vi "GTH-V2.ADC.vi"(6 "Signal Filter":T2={"Type"=enum."None", "Freq"=10000.0, "FreqB"=100.0}, 7 "Calibration_Para":dbl[][](array[numeric]), 8 "Error In":errorcluster caption="错误输入", 9 "ADC_Para":T1={"Points(X*5k)"=10, "SampleRate"=250000, "Rate"=1.0} {"Rate" min=0.01 max=100.0; "SampleRate" min=1000 max=250000 step=1000; "Points(X*5k)" min=1 max=100}, 10 "Channel":enum16{"ChanA1", "ChanA2", "ChanB1", "ChanB2"}(ring), 11 "VISA资源输入":refnum<visa-resource-name>="USB0::0x3323::0x0001::48E3845A3737::RAW") -> (0 "Error Out":errorcluster caption="错误输出", 1 "波形图":waveform(dbl)(graph), 2 "DataOut":T3={"频率"=37677.78979590854, "峰峰值"=0.1934065934065934, "均值（直流）"=-0.005379487179487172, "均方根"=0.04788898808560139, "正峰"=0.093, "反峰"=-0.10040659340659341, "幅值"=0.007320515046354128, "均方根(AC)"=0.047585883385186885} {"幅值" format="%#_8f"; "均值（直流）" format="%#_8f"}, 3 "OK?":bool=TRUE)   [LabVIEW 2012, in "Lib_UEL.ATE.lvlib" / "STM32-CoreBD.lvlib"]
uses:
  STM32-CoreBD.lvlib
  <vilib>/measure/madcrms.llb/Basic Averaged DC-RMS for 1 Chan.vi
  <vilib>/measure/NI_MAPro.lvlib
panel:
  # "Version History\nV1.0.0, 2015-8-10, GTH-V2初始版本.\nV1.1.0, 2015-10-9, ADC_Para增加Rate参数."
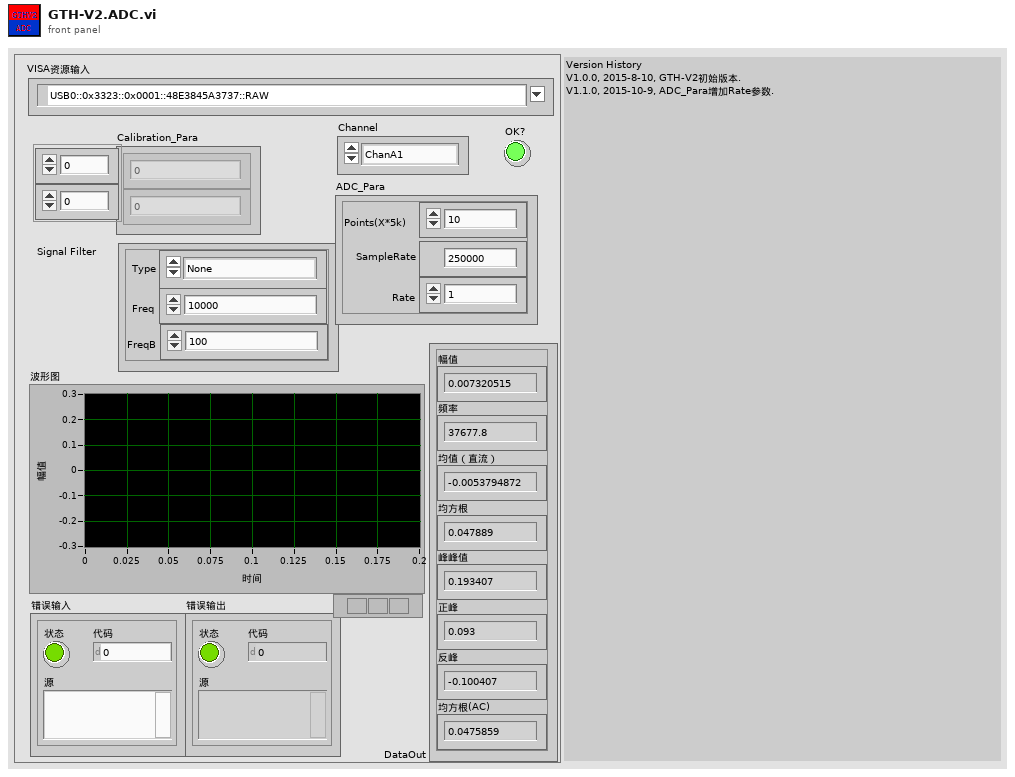
[diagram p1: front panel]
types:
  T1 = cluster{"Points(X*5k)":u8, "SampleRate":u32, "Rate":dbl}
  T2 = cluster{"Type":enum16{"None", "Low Pass", "High Pass", "Band Pass"}, "Freq":dbl, "FreqB":dbl}
  T3 = cluster{"频率":dbl, "峰峰值":dbl, "均值（直流）":dbl, "均方根":dbl, "正峰":dbl, "反峰":dbl, "幅值":dbl, "均方根(AC)":dbl}
  T4 = enum16{"Read_Version", "Read_PID", "Read_CalibrationInfo", "Read_C_Value_ADC_ChanA", "Read_C_Value_ADC_ChanB", "Read_C_Value_Current", "Read_C_Value_DAC", "Write_CalibrationInfo", "Write_C_Value_ADC_ChanA", "Write_C_Value_ADC_ChanB", "Write_C_Value_Current", "Write_C_Value_DAC"}
  T5 = enum16{"None", "Low Pass", "High Pass", "Band Pass"}
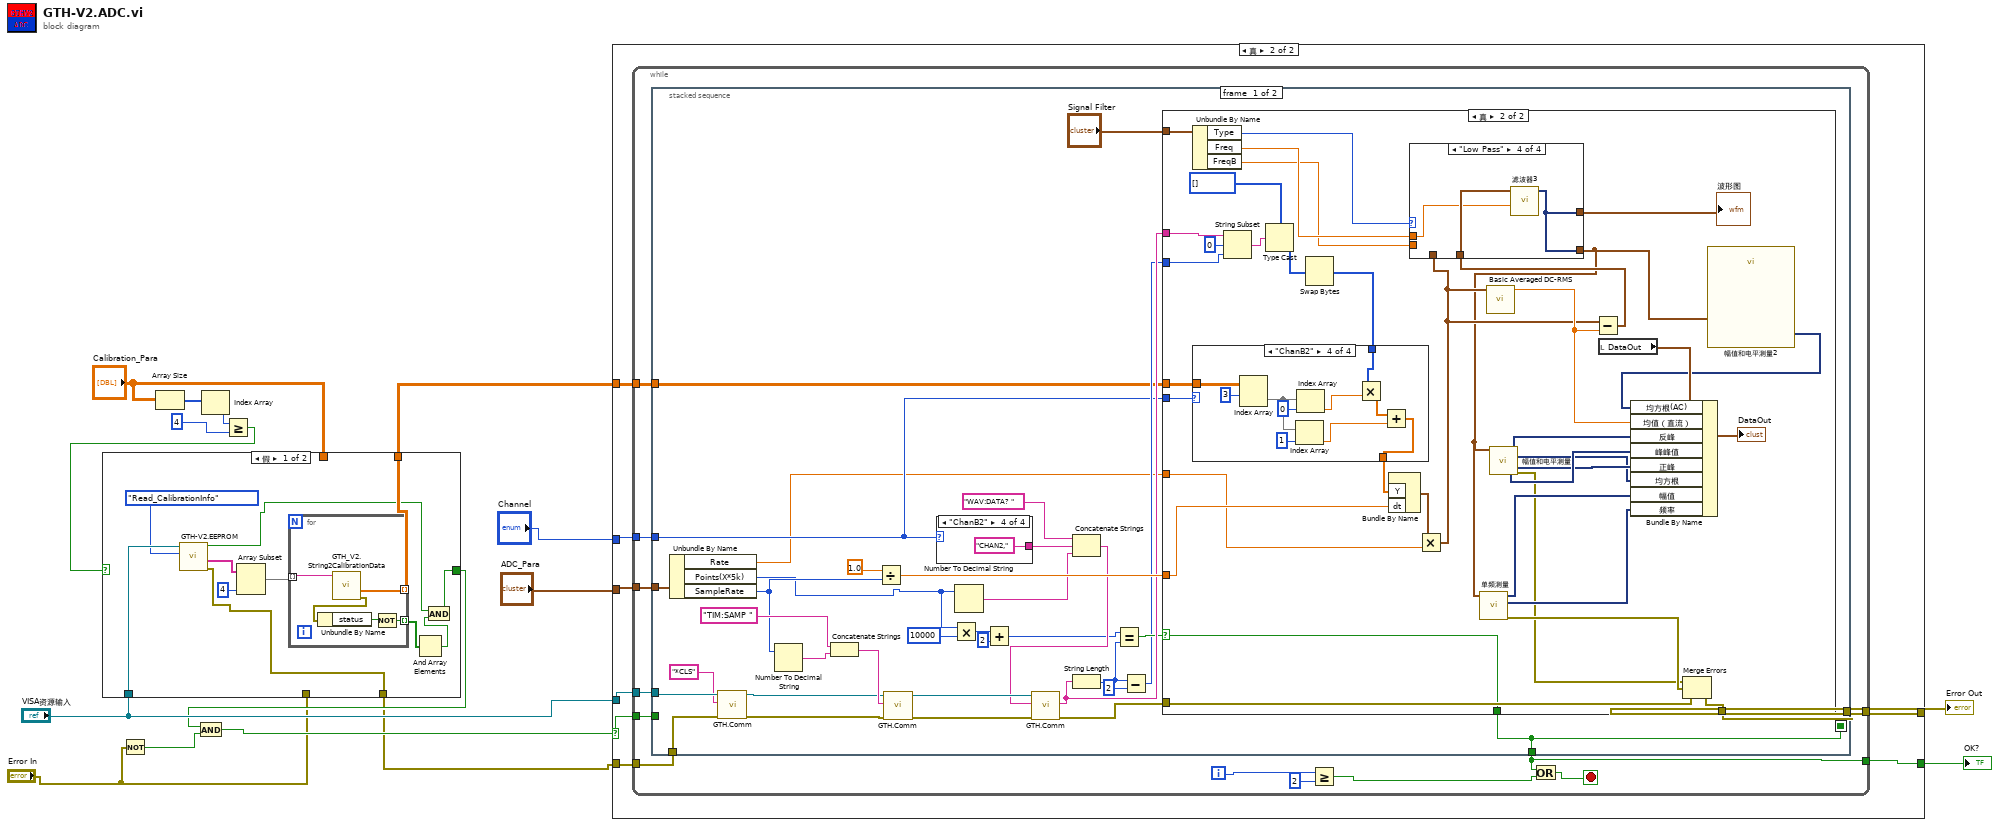
[diagram p0: block diagram]
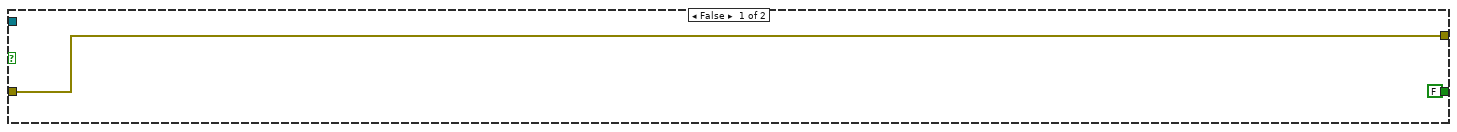
[diagram p3: hidden frame]
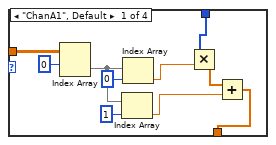
[diagram p5: hidden frame]
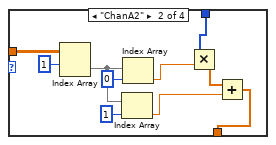
[diagram p6: hidden frame]
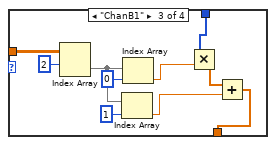
[diagram p7: hidden frame]
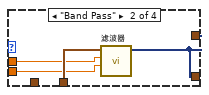
[diagram p9: hidden frame]
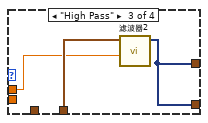
[diagram p10: hidden frame]
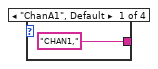
[diagram p11: hidden frame]
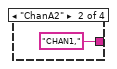
[diagram p12: hidden frame]
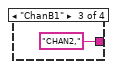
[diagram p13: hidden frame]
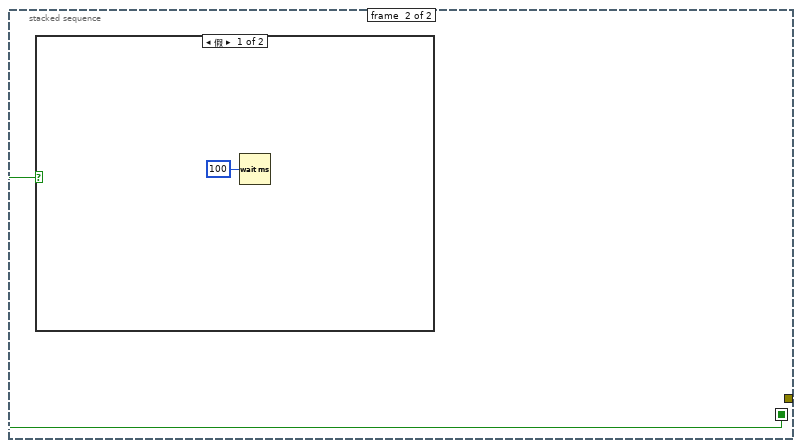
[diagram p14: hidden frame]
diagram:
  n1 = Not(x="Error In") -> (.not. x?=w10:bool)
  n2 = Array Size(array="Calibration_Para") -> (size(s)=w6:i32[])
  n3 = Index Array(array=w6) -> (element=w5:i32)  [unwired: 1 in]
  n4 = Greater Or Equal?(x=w5, y=4) -> (x >= y?=w4:bool)
  n5 = case shown="假" w4 {
    selector: w4 -> [_ w34]
    tunnel: [w22 w35] -> w9
    tunnel: "Calibration_Para" -> [_ w35]
    tunnel: "VISA资源输入" -> [w27 _]
    tunnel: [w20 w34] -> w3
    tunnel: [w19 w33] -> w2
    tunnel: "Error In" -> [_ w33]
    frame False {
      n6 = call "GTH-V2.EEPROM.vi"("CMD"=T4."Read_CalibrationInfo", "VISA资源输入"=w27) -> ("Error Out"=w19:errorcluster, "Calibration_Value_Out"=w25:string[], "OK?"=w21:bool)  [unwired: 6 in, 1 out]
      n7 = Array Subset(array=w25, length=4 ("长度")) -> (w23:string[])  [unwired: 1 in]
      n8 = for {
        tunnel: w23 -> [w32] mode=indexing
        tunnel: [w31] -> w22 mode=indexing
        tunnel: [w28] -> w18 mode=indexing
        n9 = call "GTH_V2.String2CalibrationData.vi"("String"=w32) -> ("错误输出"=w29:errorcluster, "Para"=w31:dbl[])  [unwired: 5 in, 4 out]
        n10 = Unbundle By Name(w29) -> ("status"=w30:bool)
        n11 = Not(x=w30) -> (.not. x?=w28:bool)
      }
      n12 = And Array Elements(Boolean array=w18) -> (logical AND=w17:bool)
      n13 = And(x=w21, y=w17) -> (x .and. y?=w20:bool)
    }
    frame True {
    }
  }
  n14 = And(x=w3, y=w10) -> (x .and. y?=w12:bool)
  n15 = case shown="真" w12 {
    selector: w12 -> [_ w43]
    tunnel: [w36 w45] -> w16
    tunnel: "VISA资源输入" -> [_ w44]
    tunnel: [FALSE w42] -> w15
    tunnel: "ADC_Para" -> [_ w41]
    tunnel: "Channel" -> [_ w40]
    tunnel: w2 -> [w36 w38]
    tunnel: w9 -> [_ w39]
    frame False {
    }
    frame True {
      n16 = while {
        tunnel: [w54] -> w45
        tunnel: w44 -> [w57]
        tunnel: w43 -> [w56]
        tunnel: [w50] -> w42
        tunnel: w41 -> [w49]
        tunnel: w40 -> [w48]
        tunnel: w39 -> [w47]
        tunnel: w38 -> [w46]
        i -> [w53]
        stop <- w55 stop-if-true
        n17 = stacked-sequence {
          seq-local: [w66 _] -> [_ w186]
          tunnel: w57 -> [w88 _]
          tunnel: w56 -> [_ _]
          tunnel: [w67 _] -> w54
          tunnel: [w66 _] -> w50
          tunnel: w49 -> [w64 _]
          tunnel: w48 -> [w61 _]
          tunnel: w47 -> [w60 _]
          tunnel: w46 -> [w59 _]
          frame #0 {
            n18 = Unbundle By Name(w64) -> ("Rate"=w58:dbl, "Points(X*5k)"=w62:u8, "SampleRate"=w63:u32)
            n19 = call "GTH.Comm.vi"("Error In"=w59, "SCPI CMD"="*CLS" ("字符串"), "USB Port In"=w88) -> ("Error Out"=w82:errorcluster, "USB Port Out"=w83:refnum<visa-resource-name>)  [unwired: 3 in, 4 out]
            n20 = Number To Decimal String(number=w63) -> (decimal integer string=w85:string)  [unwired: 1 in]
            n21 = Concatenate Strings("TIM:SAMP " ("字符串"), w85) -> (w84:string)
            n22 = Divide(x=1.0 ("y"), y=w63) -> (x/y=w89:dbl)
            n23 = call "GTH.Comm.vi"("Error In"=w82, "SCPI CMD"=w84, "USB Port In"=w83) -> ("Error Out"=w79:errorcluster, "USB Port Out"=w80:refnum<visa-resource-name>)  [unwired: 3 in, 4 out]
            n24 = case shown="\"ChanB2\"" w61 {
              tunnel: ["CHAN1," ("字符串") "CHAN1," ("字符串") "CHAN2," ("字符串") "CHAN2," ("字符串")] -> w91
              frame "ChanA1", Default {
              }
              frame "ChanA2" {
              }
              frame "ChanB1" {
              }
              frame "ChanB2" {
              }
            }
            n25 = Multiply(x=w62, y=u32 10000) -> (x*y=w75:u32)
            n26 = Number To Decimal String(number=w62) -> (decimal integer string=w81:string)  [unwired: 1 in]
            n27 = Add(x=w75, y=u32 2) -> (x+y=w72:u32)
            n28 = Concatenate Strings("WAV:DATA? " ("字符串"), w91, w81) -> (w78:string)
            n29 = call "GTH.Comm.vi"("Error In"=w79, "SCPI CMD"=w78, "USB Port In"=w80) -> ("Error Out"=w77:errorcluster, "Return"=w73:string)  [unwired: 3 in, 4 out]
            n30 = String Length(string=w73) -> (length=w70:i32)
            n31 = Equal?(x=w72, y=w70) -> (x = y?=w71:bool)
            n32 = Subtract(x=w70, y=2) -> (x-y=w68:i32)
            n33 = case shown="真" w71 {
              selector: w71 -> [w93 w115]
              tunnel: w89 -> [_ w128]
              tunnel: [w94 w122] -> w67
              tunnel: w77 -> [w94 w120]
              tunnel: w73 -> [_ w118]
              tunnel: w68 -> [_ w116]
              tunnel: [w93 w115] -> w66
              tunnel: "Signal Filter" -> [_ w108]
              tunnel: w61 -> [_ w103]
              tunnel: w60 -> [_ w102]
              tunnel: w58 -> [_ w99]
              frame False {
              }
              frame True {
                n34 = Unbundle By Name(w108) -> ("Type"=w107:T5, "Freq"=w104:dbl, "FreqB"=w95:dbl)
                n35 = String Subset(string=w118, offset (0)=0 ("偏移量(0)"), length (rest)=w116) -> (substring=w119:string)
                n36 = Type Cast(type=u16[] [], x=w119) -> (*(type *) &x=w129:u16[])
                n37 = Swap Bytes(anything=w129) -> (byte swapped=w100:u16[])
                n38 = case shown="\"ChanB2\"" w103 {
                  tunnel: w102 -> [w140 w150 w160 w170]
                  tunnel: w100 -> [w138 w148 w158 w168]
                  tunnel: [w136 w146 w156 w166] -> w101
                  frame "ChanA1", Default {
                    n39 = Index Array(array=w140, index (row)=0 ("索引")) -> (element=w135:dbl[])  [unwired: 1 in]
                    n40 = Index Array(array=w135, index=1 ("索引")) -> (element=w131:dbl)
                    n41 = Index Array(array=w135, index=0 ("索引")) -> (element=w132:dbl)
                    n42 = Multiply(x=w138, y=w132) -> (x*y=w137:dbl[])
                    n43 = Add(x=w137, y=w131) -> (x+y=w136:dbl[])
                  }
                  frame "ChanA2" {
                    n44 = Index Array(array=w150, index (row)=1 ("索引")) -> (element=w145:dbl[])  [unwired: 1 in]
                    n45 = Index Array(array=w145, index=1 ("索引")) -> (element=w141:dbl)
                    n46 = Index Array(array=w145, index=0 ("索引")) -> (element=w142:dbl)
                    n47 = Multiply(x=w148, y=w142) -> (x*y=w147:dbl[])
                    n48 = Add(x=w147, y=w141) -> (x+y=w146:dbl[])
                  }
                  frame "ChanB1" {
                    n49 = Index Array(array=w160, index (row)=2 ("索引")) -> (element=w155:dbl[])  [unwired: 1 in]
                    n50 = Index Array(array=w155, index=1 ("索引")) -> (element=w151:dbl)
                    n51 = Index Array(array=w155, index=0 ("索引")) -> (element=w152:dbl)
                    n52 = Multiply(x=w158, y=w152) -> (x*y=w157:dbl[])
                    n53 = Add(x=w157, y=w151) -> (x+y=w156:dbl[])
                  }
                  frame "ChanB2" {
                    n54 = Index Array(array=w170, index (row)=3 ("索引")) -> (element=w165:dbl[])  [unwired: 1 in]
                    n55 = Index Array(array=w165, index=1 ("索引")) -> (element=w161:dbl)
                    n56 = Index Array(array=w165, index=0 ("索引")) -> (element=w162:dbl)
                    n57 = Multiply(x=w168, y=w162) -> (x*y=w167:dbl[])
                    n58 = Add(x=w167, y=w161) -> (x+y=w166:dbl[])
                  }
                }
                n59 = Bundle By Name("Y"=w101, "dt"=w128) -> (w98:waveform(dbl))  [unwired: 1 in]
                n60 = Multiply(x=w98, y=w99) -> (x*y=w97:waveform(dbl))
                n61 = call-poly <vilib>:"Basic Averaged DC-RMS.vi"("signal in"=w97) -> ("DC value"=w121:dbl)  [unwired: 7 in, 3 out]
                n62 = Subtract(x=w97, y=w121) -> (x-y=w105:waveform(dbl))
                n63 = case shown="\"Low Pass\"" w107 {
                  tunnel: [w171 w174 w176 w179] -> w106
                  tunnel: w97 -> [w171 _ _ _]
                  tunnel: [w171 w174 w176 w179] -> w96
                  tunnel: w105 -> [_ w175 w178 w181]
                  tunnel: w104 -> [_ w173 w177 w180]
                  tunnel: w95 -> [_ w172 _ _]
                  frame "None", Default {
                  }
                  frame "Band Pass" {
                    n64 = call "滤波器"("Lower Cut-Off"=w172, "Upper Cut-Off"=w173, "Signal"=w175) -> ("Filtered Signal"=w174:dynamicdata)  [unwired: 7 in, 1 out]
                  }
                  frame "High Pass" {
                    n65 = call "滤波器2"("Lower Cut-Off"=w177, "Signal"=w178) -> ("Filtered Signal"=w176:dynamicdata)  [unwired: 8 in, 1 out]
                  }
                  frame "Low Pass" {
                    n66 = call "滤波器3"("Lower Cut-Off"=w180, "Signal"=w181) -> ("Filtered Signal"=w179:dynamicdata)  [unwired: 8 in, 1 out]
                  }
                }
                "波形图" <- w106
                n67 = call "单频测量"("Signals"=w96) -> ("error out"=w127:errorcluster, "Frequency"=w123:dynamicdata, "Amplitude"=w124:dynamicdata)  [unwired: 8 in]
                n68 = call "幅值和电平测量"("Signals"=w96) -> ("RMS"=w111:dynamicdata, "Negative Peak"=w114:dynamicdata, "Positive Peak"=w112:dynamicdata, "Peak to Peak"=w113:dynamicdata, "error out"=w109:errorcluster)  [unwired: 10 in]
                n69 = local read "DataOut"() -> (w125:T3)
                n70 = Merge Errors(w109, w127, w120) -> (w122:errorcluster)
                n71 = call "幅值和电平测量2"("Signals"=w96) -> ("RMS"=w110:dynamicdata)  [unwired: 13 in, 1 out]
                n72 = Bundle By Name(cluster=w125, "均方根(AC)"=w110, "均值（直流）"=w121, "反峰"=w114, "峰峰值"=w113, "正峰"=w112, "均方根"=w111, "幅值"=w124, "频率"=w123) -> (→"DataOut":T3)
              }
            }
          }
          frame #1 {
            n73 = case shown="假" w186 {
              frame False {
                n74 = Wait (ms)(milliseconds to wait=u32 100 ("等待时间（毫秒）")) -> ()  [unwired: 1 out]
              }
              frame True {
              }
            }
          }
        }
        n75 = Greater Or Equal?(x=w53, y=2) -> (x >= y?=w51:bool)
        n76 = Or(x=w50, y=w51) -> (x .or. y?=w55:bool)
      }
    }
  }
  "Error Out" <- w16
  "OK?" <- w15
